vi "Send CMD.vi"(8 "error in":errorcluster, 10 "CMD In":string, 11 "Vaisala in":refnum<class "Vaisala.lvclass">=refnum) -> (0 "error out":errorcluster, 3 "Vaisala out":refnum<class "Vaisala.lvclass">)   [LabVIEW 2015, in "Vaisala Library.lvlib" / "Vaisala.lvclass"]
uses:
  Vaisala.lvclass
  <vilib>/MSR Consulting, LLC/General Reuse/Session APIs/Serial/Serial Session.lvclass
  <vilib>/MSR Consulting, LLC/General Reuse/Session APIs/Serial/Public/Get Data/Get String.vi
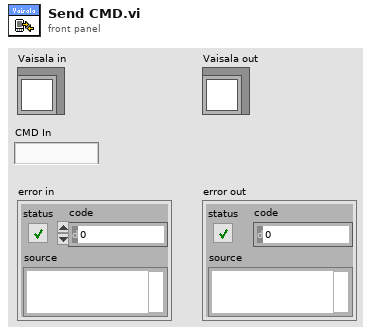
[diagram p1: front panel]
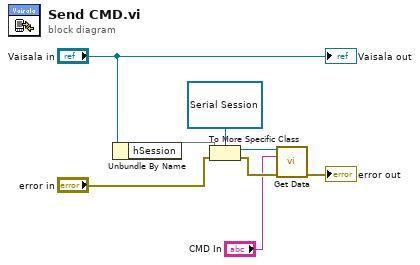
[diagram p0: block diagram]
diagram:
  n1 = Unbundle By Name("Vaisala in") -> ("hSession"=w6)
  n2 = To More Specific Class(target class=refnum<data-value> refnum, reference=w6, error in="error in") -> (specific class reference=w2:refnum<data-value>, error out=w4:errorcluster)
  n3 = call-poly <vilib>:"Get Data.vi"("Session Handle in"=w2, "CMD"="CMD In", "error in"=w4) -> ("error out"=→"error out":errorcluster)  [unwired: 10 in, 2 out]
  "Vaisala out" <- "Vaisala in"
